vi "Sucesion 1.vi"() -> ()   [LabVIEW 2017]
panel:
  out "Iteración":i32
  out "Número":i64
  # "SUCESIÓN 1"
  # "CECILIA NUÑEZ\n    11541028"
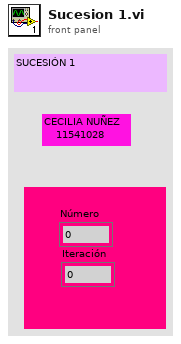
[diagram p1: front panel]
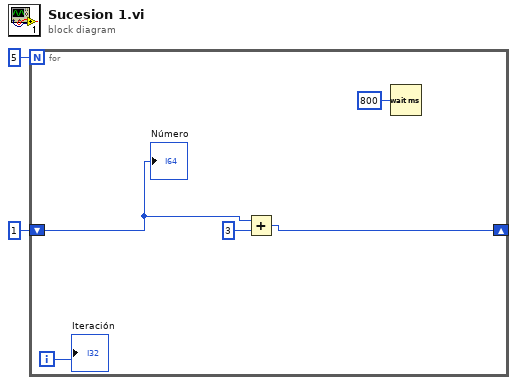
[diagram p0: block diagram]
diagram:
  n1 = for {
    N: 5 -> [_]
    shift-right: [w4] -> _
    shift-left: i64 1 -> [w3]
    i -> [w6]
    n2 = Add(x=w3, y=i64 3) -> (x+y=w4:i64)
    n3 = Wait (ms)(milliseconds to wait=u32 800) -> ()  [unwired: 1 out]
    "Iteración" <- w6
    "Número" <- w3
  }
